vi "Main.vi"() -> ()   [LabVIEW 2017]
panel:
  out "sortie d'erreur":errorcluster
  in  "Error In":errorcluster caption="entrée d'erreur (pas d'erreur)"
  in  "Port":u16=3000
  in  "TCP Address":string="192.168.1.4"
  in  "Cluster":T1
  out "octets écrits":i32
  in  "Bouton Stop":bool
  # "SainSmart iMatic RJ45 TCP/IP Remote Control Board for 16-Ch Relay"
  # "Relais 1"
  # "Moteur"
  # "Pompe"
  # "EV 1"
  # "EV 2"
  # "EV 3"
  # "EV 4"
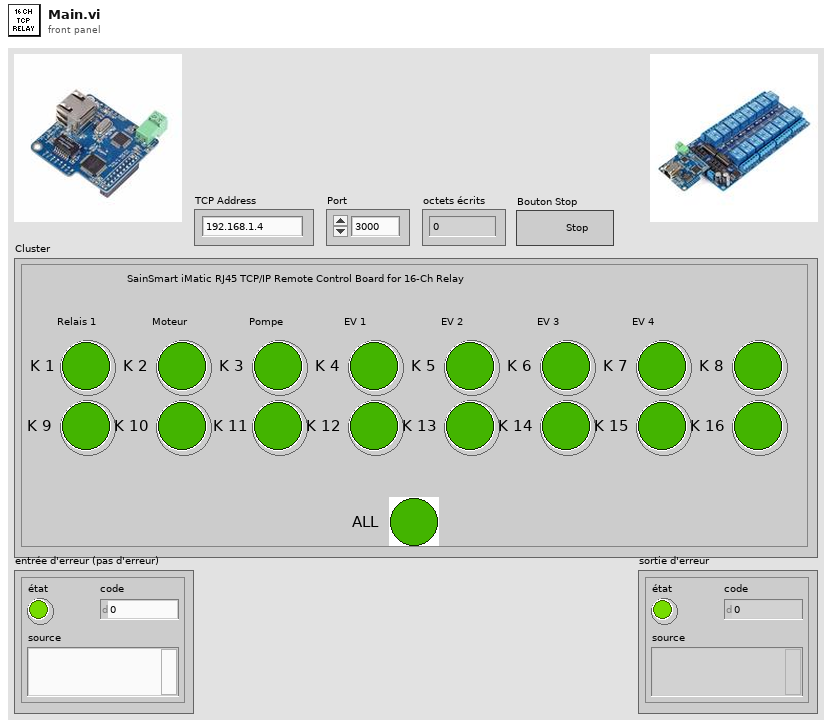
[diagram p1: front panel]
types:
  T1 = cluster{"K 1":bool, "K 2":bool, "K 3":bool, "K 4":bool, "K 5":bool, "K 6":bool, "K 7":bool, "K 8":bool, "K 9":bool, "K 10":bool, "K 11":bool, "K 12":bool, "K 13":bool, "K 14":bool, "K 15":bool, "K 16":bool, "ALL":bool}
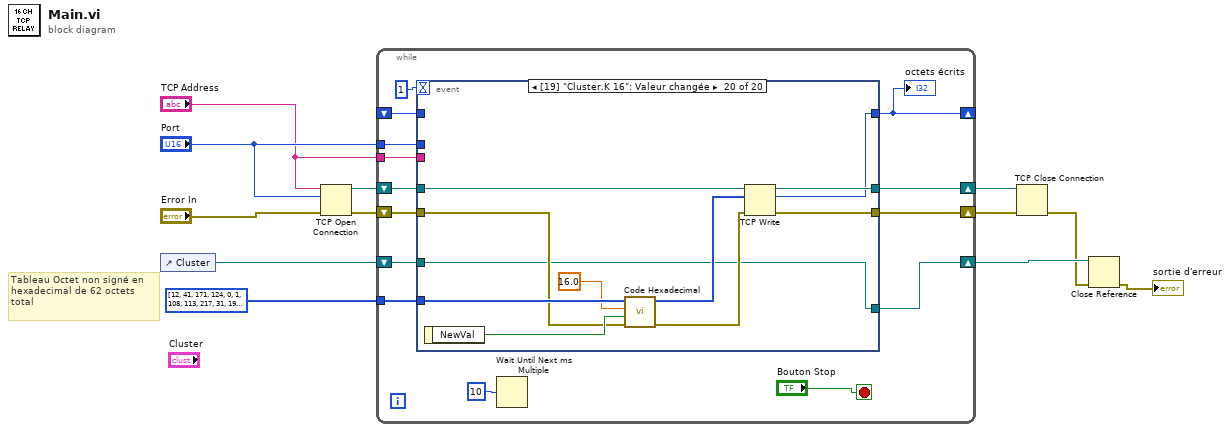
[diagram p0: block diagram]
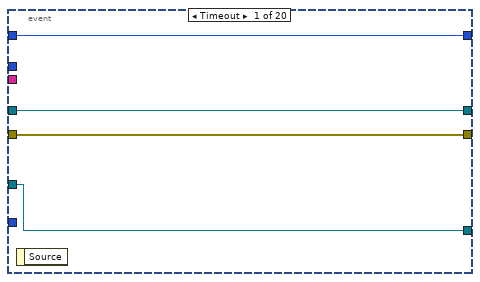
[diagram p2: hidden frame]
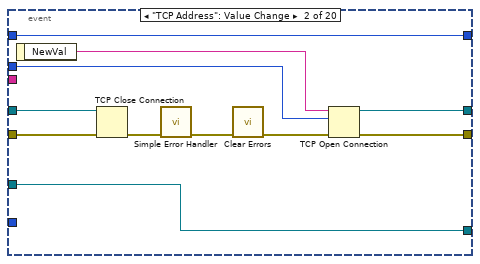
[diagram p3: hidden frame]
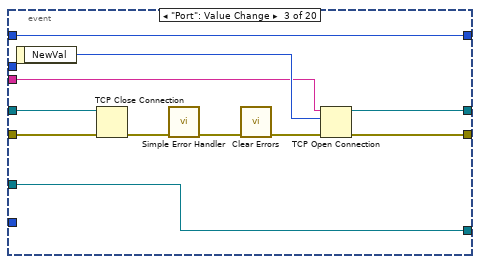
[diagram p4: hidden frame]
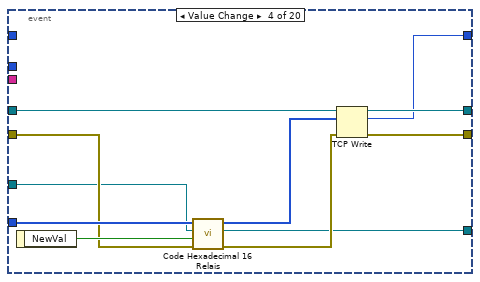
[diagram p5: hidden frame]
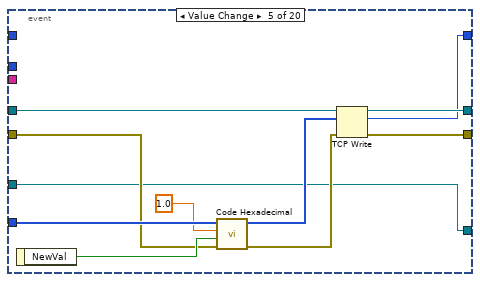
[diagram p6: hidden frame]
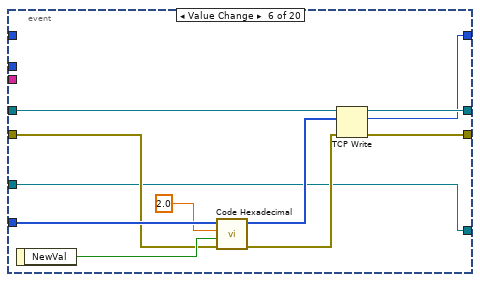
[diagram p7: hidden frame]
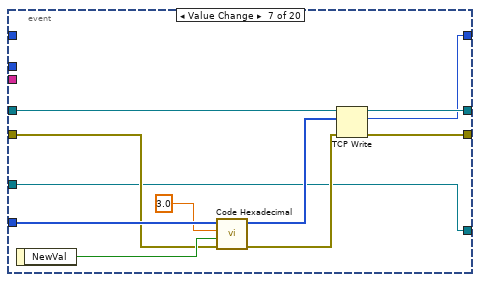
[diagram p8: hidden frame]
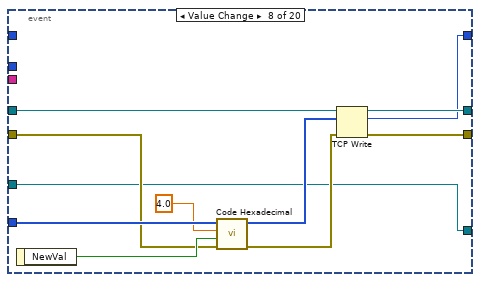
[diagram p9: hidden frame]
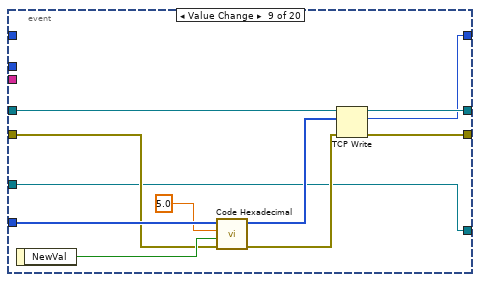
[diagram p10: hidden frame]
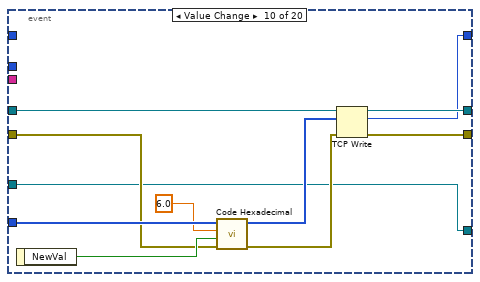
[diagram p11: hidden frame]
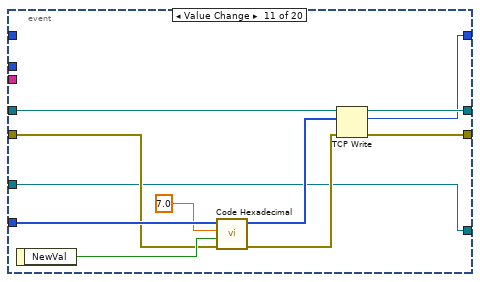
[diagram p12: hidden frame]
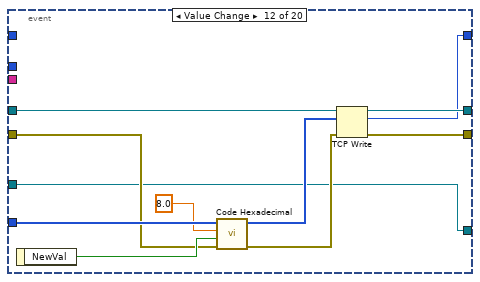
[diagram p13: hidden frame]
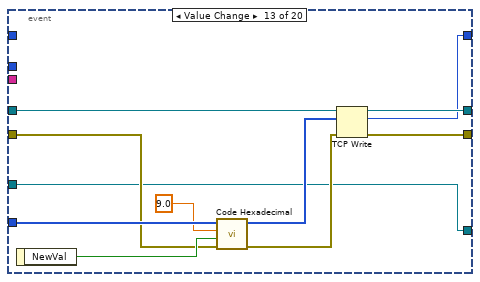
[diagram p14: hidden frame]
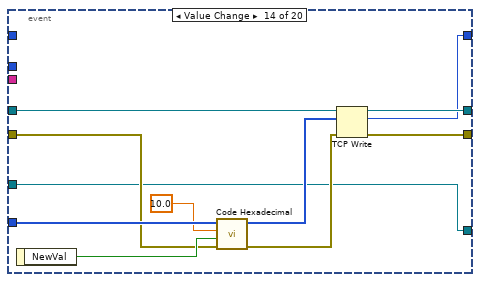
[diagram p15: hidden frame]
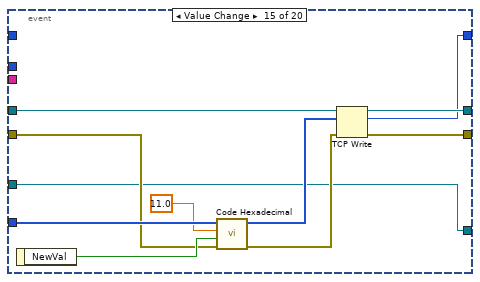
[diagram p16: hidden frame]
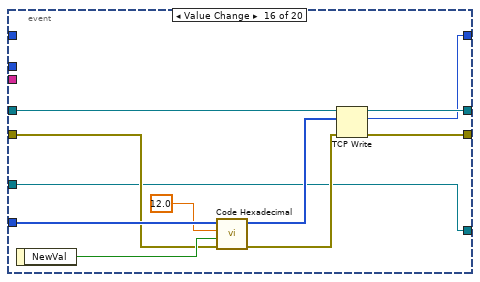
[diagram p17: hidden frame]
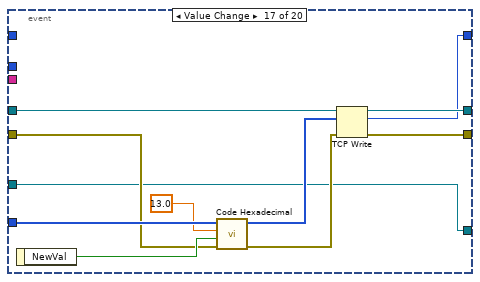
[diagram p18: hidden frame]
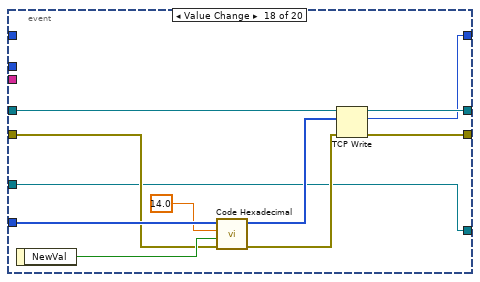
[diagram p19: hidden frame]
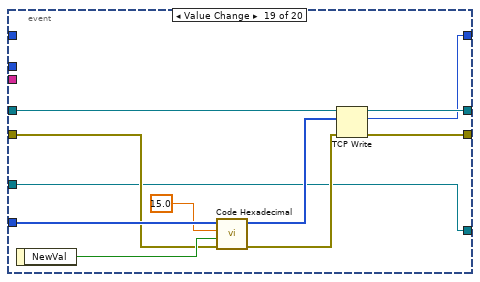
[diagram p20: hidden frame]
diagram:
  # "Tableau Octet non signé en hexadecimal de 62 octets total"
  n1 = control-ref of="Cluster"() -> (w5:refnum<vi>)
  n2 = TCP Open Connection(address="TCP Address", remote port or service name="Port", error in (no error)="Error In") -> (connection ID=w11:refnum<k5>, error out=w10:errorcluster)  [unwired: 2 in]
  n3 = while {
    shift-right: [w20] -> w12
    shift-left: w11 -> [w23]
    shift-right: [w15] -> w4
    shift-left: w10 -> [w22]
    tunnel: "Port" -> [w21]
    tunnel: "TCP Address" -> [w19]
    tunnel: u8[] [12, 41, 171, 124, 0, 1, 108, 113, 217, 31, 198, 65, 8, 0, 69, 0, 0, 48, 111, 152, 64, 0, 128, 6, 7, 193, 192, 168, 1, 26, 192, 168, 1, 4, 214, 0, 11, 184, 114, 220, 20, 37, 193, 253, 187, 189, 80, 24, 250, 216, 223, 153, 0, 0, 88, 1] ("tableau sans le sous-tableau") -> [w18]
    shift-right: [w17] -> _
    shift-left: _ -> [w16]
    shift-right: [w13] -> w3
    shift-left: w5 -> [w14]
    stop <- "Bouton Stop" stop-if-true
    n4 = event shown="[19] \"Cluster.K 16\": Valeur changée" {
      selector: _ -> [_ _ _ _ _ _ _ _ _ _ _ _ _ _ _ _ _ _ _ _]
      dyn-events: _ -> [_ _ _ _ _ _ _ _ _ _ _ _ _ _ _ _ _ _ _ _]
      timeout: 1 -> [_ _ _ _ _ _ _ _ _ _ _ _ _ _ _ _ _ _ _ _]
      tunnel: w23 -> [w30 w41 w52 w63 w65 w76 w87 w98 w109 w120 w131 w142 w153 w164 w175 w186 w197 w208 w219 w230]
      tunnel: w22 -> [w29 w40 w51 w55 w66 w77 w88 w99 w110 w121 w132 w143 w154 w165 w176 w187 w198 w209 w220 w231]
      tunnel: w21 -> [_ w38 _ _ _ _ _ _ _ _ _ _ _ _ _ _ _ _ _ _]
      tunnel: [w30 w37 w50 w62 w73 w84 w95 w106 w117 w128 w139 w150 w161 w172 w183 w194 w205 w216 w227 w238] -> w20
      tunnel: [w29 w36 w49 w61 w74 w85 w96 w107 w118 w129 w140 w151 w162 w173 w184 w195 w206 w217 w228 w239] -> w15
      tunnel: w19 -> [_ _ w47 _ _ _ _ _ _ _ _ _ _ _ _ _ _ _ _ _]
      tunnel: w18 -> [_ _ _ w58 w70 w81 w92 w103 w114 w125 w136 w147 w158 w169 w180 w191 w202 w213 w224 w235]
      tunnel: [w28 w35 w46 w60 w72 w83 w94 w105 w116 w127 w138 w149 w160 w171 w182 w193 w204 w215 w226 w237] -> w17
      tunnel: w16 -> [w28 w35 w46 _ _ _ _ _ _ _ _ _ _ _ _ _ _ _ _ _]
      tunnel: w14 -> [w27 w31 w42 w54 w64 w75 w86 w97 w108 w119 w130 w141 w152 w163 w174 w185 w196 w207 w218 w229]
      tunnel: [w27 w31 w42 w53 w64 w75 w86 w97 w108 w119 w130 w141 w152 w163 w174 w185 w196 w207 w218 w229] -> w13
      event Timeout {
        n5 = event-data() -> ()  [unwired: 1 in, 1 out]
      }
      event "TCP Address": Value Change {
        n6 = event-data() -> ("NewVal"=w39:string)  [unwired: 1 in]
        n7 = TCP Close Connection(connection ID=w41, error in (no error)=w40) -> (error out=w33:errorcluster)  [unwired: 1 in, 1 out]
        n8 = call <vilib>:"Simple Error Handler.vi"("error in (no error)"=w33) -> ("error out"=w32:errorcluster)  [unwired: 4 in, 4 out]
        n9 = call <vilib>:"Clear Errors.vi"("error in (no error)"=w32) -> ("error out"=w34:errorcluster)  [unwired: 5 in, 1 out]
        n10 = TCP Open Connection(address=w39, remote port or service name=w38, error in (no error)=w34) -> (connection ID=w37:refnum<k5>, error out=w36:errorcluster)  [unwired: 2 in]
      }
      event "Port": Value Change {
        n11 = event-data() -> ("NewVal"=w48:u16)  [unwired: 1 in]
        n12 = TCP Close Connection(connection ID=w52, error in (no error)=w51) -> (error out=w44:errorcluster)  [unwired: 1 in, 1 out]
        n13 = call <vilib>:"Simple Error Handler.vi"("error in (no error)"=w44) -> ("error out"=w43:errorcluster)  [unwired: 4 in, 4 out]
        n14 = call <vilib>:"Clear Errors.vi"("error in (no error)"=w43) -> ("error out"=w45:errorcluster)  [unwired: 5 in, 1 out]
        n15 = TCP Open Connection(address=w47, remote port or service name=w48, error in (no error)=w45) -> (connection ID=w50:refnum<k5>, error out=w49:errorcluster)  [unwired: 2 in]
      }
      event "Cluster.ALL": Value Change {
        n16 = event-data() -> ("NewVal"=w59:bool)  [unwired: 1 in]
        n17 = call "Code Hexadecimal 16 Relais.vi"("Error In"=w55, "Etat"=w59, "référence"=w54, "tableau code"=w58) -> ("Error Out"=w56:errorcluster, "référence en sortie"=w53:refnum<vi>, "tableau en sortie"=w57:u8[])  [unwired: 5 in]
        n18 = TCP Write(connection ID=w63, data in=w57, error in (no error)=w56) -> (connection ID out=w62:refnum<k5>, bytes written=w60:i32, error out=w61:errorcluster)  [unwired: 1 in]
      }
      event "Cluster.K 1": Value Change {
        n19 = event-data() -> ("NewVal"=w68:bool)  [unwired: 1 in]
        n20 = call "Code Hexadecimal.vi"("Error In"=w66, "Etat"=w68, "Numéro Relais"=1.0, "tableau code"=w70) -> ("Error Out"=w71:errorcluster, "tableau en sortie"=w69:u8[])  [unwired: 6 in]
        n21 = TCP Write(connection ID=w65, data in=w69, error in (no error)=w71) -> (connection ID out=w73:refnum<k5>, bytes written=w72:i32, error out=w74:errorcluster)  [unwired: 1 in]
      }
      event "Cluster.K 2": Value Change {
        n22 = event-data() -> ("NewVal"=w79:bool)  [unwired: 1 in]
        n23 = call "Code Hexadecimal.vi"("Error In"=w77, "Etat"=w79, "Numéro Relais"=2.0, "tableau code"=w81) -> ("Error Out"=w82:errorcluster, "tableau en sortie"=w80:u8[])  [unwired: 6 in]
        n24 = TCP Write(connection ID=w76, data in=w80, error in (no error)=w82) -> (connection ID out=w84:refnum<k5>, bytes written=w83:i32, error out=w85:errorcluster)  [unwired: 1 in]
      }
      event "Cluster.K 3": Value Change {
        n25 = event-data() -> ("NewVal"=w90:bool)  [unwired: 1 in]
        n26 = call "Code Hexadecimal.vi"("Error In"=w88, "Etat"=w90, "Numéro Relais"=3.0, "tableau code"=w92) -> ("Error Out"=w93:errorcluster, "tableau en sortie"=w91:u8[])  [unwired: 6 in]
        n27 = TCP Write(connection ID=w87, data in=w91, error in (no error)=w93) -> (connection ID out=w95:refnum<k5>, bytes written=w94:i32, error out=w96:errorcluster)  [unwired: 1 in]
      }
      event "Cluster.K 4": Value Change {
        n28 = event-data() -> ("NewVal"=w101:bool)  [unwired: 1 in]
        n29 = call "Code Hexadecimal.vi"("Error In"=w99, "Etat"=w101, "Numéro Relais"=4.0, "tableau code"=w103) -> ("Error Out"=w104:errorcluster, "tableau en sortie"=w102:u8[])  [unwired: 6 in]
        n30 = TCP Write(connection ID=w98, data in=w102, error in (no error)=w104) -> (connection ID out=w106:refnum<k5>, bytes written=w105:i32, error out=w107:errorcluster)  [unwired: 1 in]
      }
      event "Cluster.K 5": Value Change {
        n31 = event-data() -> ("NewVal"=w112:bool)  [unwired: 1 in]
        n32 = call "Code Hexadecimal.vi"("Error In"=w110, "Etat"=w112, "Numéro Relais"=5.0, "tableau code"=w114) -> ("Error Out"=w115:errorcluster, "tableau en sortie"=w113:u8[])  [unwired: 6 in]
        n33 = TCP Write(connection ID=w109, data in=w113, error in (no error)=w115) -> (connection ID out=w117:refnum<k5>, bytes written=w116:i32, error out=w118:errorcluster)  [unwired: 1 in]
      }
      event "Cluster.K 6": Value Change {
        n34 = event-data() -> ("NewVal"=w123:bool)  [unwired: 1 in]
        n35 = call "Code Hexadecimal.vi"("Error In"=w121, "Etat"=w123, "Numéro Relais"=6.0, "tableau code"=w125) -> ("Error Out"=w126:errorcluster, "tableau en sortie"=w124:u8[])  [unwired: 6 in]
        n36 = TCP Write(connection ID=w120, data in=w124, error in (no error)=w126) -> (connection ID out=w128:refnum<k5>, bytes written=w127:i32, error out=w129:errorcluster)  [unwired: 1 in]
      }
      event "Cluster.K 7": Value Change {
        n37 = event-data() -> ("NewVal"=w134:bool)  [unwired: 1 in]
        n38 = call "Code Hexadecimal.vi"("Error In"=w132, "Etat"=w134, "Numéro Relais"=7.0, "tableau code"=w136) -> ("Error Out"=w137:errorcluster, "tableau en sortie"=w135:u8[])  [unwired: 6 in]
        n39 = TCP Write(connection ID=w131, data in=w135, error in (no error)=w137) -> (connection ID out=w139:refnum<k5>, bytes written=w138:i32, error out=w140:errorcluster)  [unwired: 1 in]
      }
      event "Cluster.K 8": Value Change {
        n40 = event-data() -> ("NewVal"=w145:bool)  [unwired: 1 in]
        n41 = call "Code Hexadecimal.vi"("Error In"=w143, "Etat"=w145, "Numéro Relais"=8.0, "tableau code"=w147) -> ("Error Out"=w148:errorcluster, "tableau en sortie"=w146:u8[])  [unwired: 6 in]
        n42 = TCP Write(connection ID=w142, data in=w146, error in (no error)=w148) -> (connection ID out=w150:refnum<k5>, bytes written=w149:i32, error out=w151:errorcluster)  [unwired: 1 in]
      }
      event "Cluster.K 9": Value Change {
        n43 = event-data() -> ("NewVal"=w156:bool)  [unwired: 1 in]
        n44 = call "Code Hexadecimal.vi"("Error In"=w154, "Etat"=w156, "Numéro Relais"=9.0, "tableau code"=w158) -> ("Error Out"=w159:errorcluster, "tableau en sortie"=w157:u8[])  [unwired: 6 in]
        n45 = TCP Write(connection ID=w153, data in=w157, error in (no error)=w159) -> (connection ID out=w161:refnum<k5>, bytes written=w160:i32, error out=w162:errorcluster)  [unwired: 1 in]
      }
      event "Cluster.K 10": Value Change {
        n46 = event-data() -> ("NewVal"=w167:bool)  [unwired: 1 in]
        n47 = call "Code Hexadecimal.vi"("Error In"=w165, "Etat"=w167, "Numéro Relais"=10.0, "tableau code"=w169) -> ("Error Out"=w170:errorcluster, "tableau en sortie"=w168:u8[])  [unwired: 6 in]
        n48 = TCP Write(connection ID=w164, data in=w168, error in (no error)=w170) -> (connection ID out=w172:refnum<k5>, bytes written=w171:i32, error out=w173:errorcluster)  [unwired: 1 in]
      }
      event "Cluster.K 11": Value Change {
        n49 = event-data() -> ("NewVal"=w178:bool)  [unwired: 1 in]
        n50 = call "Code Hexadecimal.vi"("Error In"=w176, "Etat"=w178, "Numéro Relais"=11.0, "tableau code"=w180) -> ("Error Out"=w181:errorcluster, "tableau en sortie"=w179:u8[])  [unwired: 6 in]
        n51 = TCP Write(connection ID=w175, data in=w179, error in (no error)=w181) -> (connection ID out=w183:refnum<k5>, bytes written=w182:i32, error out=w184:errorcluster)  [unwired: 1 in]
      }
      event "Cluster.K 12": Value Change {
        n52 = event-data() -> ("NewVal"=w189:bool)  [unwired: 1 in]
        n53 = call "Code Hexadecimal.vi"("Error In"=w187, "Etat"=w189, "Numéro Relais"=12.0, "tableau code"=w191) -> ("Error Out"=w192:errorcluster, "tableau en sortie"=w190:u8[])  [unwired: 6 in]
        n54 = TCP Write(connection ID=w186, data in=w190, error in (no error)=w192) -> (connection ID out=w194:refnum<k5>, bytes written=w193:i32, error out=w195:errorcluster)  [unwired: 1 in]
      }
      event "Cluster.K 13": Value Change {
        n55 = event-data() -> ("NewVal"=w200:bool)  [unwired: 1 in]
        n56 = call "Code Hexadecimal.vi"("Error In"=w198, "Etat"=w200, "Numéro Relais"=13.0, "tableau code"=w202) -> ("Error Out"=w203:errorcluster, "tableau en sortie"=w201:u8[])  [unwired: 6 in]
        n57 = TCP Write(connection ID=w197, data in=w201, error in (no error)=w203) -> (connection ID out=w205:refnum<k5>, bytes written=w204:i32, error out=w206:errorcluster)  [unwired: 1 in]
      }
      event "Cluster.K 14": Value Change {
        n58 = event-data() -> ("NewVal"=w211:bool)  [unwired: 1 in]
        n59 = call "Code Hexadecimal.vi"("Error In"=w209, "Etat"=w211, "Numéro Relais"=14.0, "tableau code"=w213) -> ("Error Out"=w214:errorcluster, "tableau en sortie"=w212:u8[])  [unwired: 6 in]
        n60 = TCP Write(connection ID=w208, data in=w212, error in (no error)=w214) -> (connection ID out=w216:refnum<k5>, bytes written=w215:i32, error out=w217:errorcluster)  [unwired: 1 in]
      }
      event "Cluster.K 15": Value Change {
        n61 = event-data() -> ("NewVal"=w222:bool)  [unwired: 1 in]
        n62 = call "Code Hexadecimal.vi"("Error In"=w220, "Etat"=w222, "Numéro Relais"=15.0, "tableau code"=w224) -> ("Error Out"=w225:errorcluster, "tableau en sortie"=w223:u8[])  [unwired: 6 in]
        n63 = TCP Write(connection ID=w219, data in=w223, error in (no error)=w225) -> (connection ID out=w227:refnum<k5>, bytes written=w226:i32, error out=w228:errorcluster)  [unwired: 1 in]
      }
      event "Cluster.K 16": Value Change {
        n64 = event-data() -> ("NewVal"=w233:bool)  [unwired: 1 in]
        n65 = call "Code Hexadecimal.vi"("Error In"=w231, "Etat"=w233, "Numéro Relais"=16.0, "tableau code"=w235) -> ("Error Out"=w236:errorcluster, "tableau en sortie"=w234:u8[])  [unwired: 6 in]
        n66 = TCP Write(connection ID=w230, data in=w234, error in (no error)=w236) -> (connection ID out=w238:refnum<k5>, bytes written=w237:i32, error out=w239:errorcluster)  [unwired: 1 in]
      }
    }
    "octets écrits" <- w17
    n67 = Wait Until Next ms Multiple(millisecond multiple=u32 10 ("n millisecondes")) -> ()  [unwired: 1 out]
  }
  n68 = TCP Close Connection(connection ID=w12, error in (no error)=w4) -> (error out=w2:errorcluster)  [unwired: 1 in, 1 out]
  n69 = Close Reference(reference=w3, error in (no error)=w2) -> (error out=→"sortie d'erreur":errorcluster)
